vi "IVC_OC200_format_data.vi"(8 "element":dbl[](array[numeric]), 11 "time":timestamp) -> (3 "waveform_array_A":waveform(dbl)[](array[waveform])=[{"t0"=timestamp(0 s since 1904-01-01), "dt"=1.0, "Y"=[]}, {"t0"=timestamp(3732035173.078092 s since 1904-01-01), "dt"=1.0, "Y"=[302.8589782714844], "attributes"=variant("NI_ChannelName"=variant(string "T1"))}])   [LabVIEW 2019]
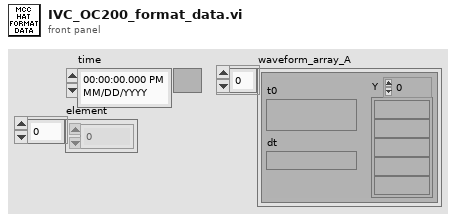
[diagram p1: front panel]
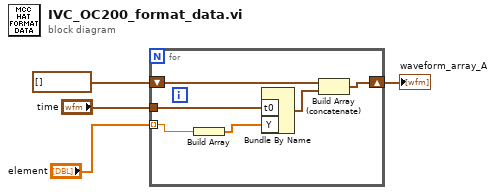
[diagram p0: block diagram]
diagram:
  n1 = for {
    tunnel: "time" -> [w9]
    shift-right: [w8] -> w4
    shift-left: waveform(dbl)[] [] -> [w10]
    tunnel: "element" -> [w6] mode=indexing
    n2 = Build Array(w6) -> (w5:dbl[])
    n3 = Bundle By Name("t0"=w9, "Y"=w5) -> (w7:waveform(dbl))  [unwired: 1 in]
    n4 = Build Array (concatenate)(w10, w7) -> (w8:waveform(dbl)[])
  }
  "waveform_array_A" <- w4
